vi "VCI_ClearBuffer.vi"(9 "CANIndex 2":u32, 10 "DevIndex 2":u32, 11 "DevType 2":u32) -> (1 "CANIndex":u32, 2 "DevIndex":u32, 3 "DevType":u32, 5 "ClearBuffer_Success？":u32)   [LabVIEW 2014]
uses:
  ControlCAN.dll
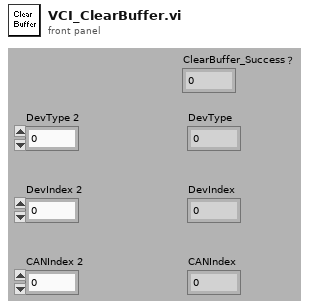
[diagram p1: front panel]
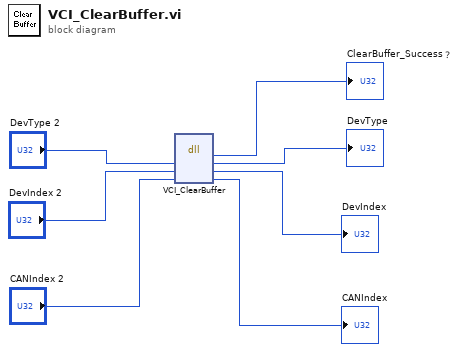
[diagram p0: block diagram]
diagram:
  n1 = dll-call lib="PTH22abs D\tDocuments\tCan总线canControlCAN.dll" fn="VCI_ClearBuffer"("DevType"="DevType 2", "DevIndex"="DevIndex 2", "CANIndex"="CANIndex 2") -> ("ClearBuffer_Success？"=→"ClearBuffer_Success？":u32, "DevType"=→"DevType":u32, "DevIndex"=→"DevIndex":u32, "CANIndex"=→"CANIndex":u32)  [unwired: 3 in, 2 out]
